vi "LJM logger process data.vi"(6 "Disable Scaling":bool, 9 "Scaling Equation":string[](array[string]), 10 "# Channels":i32, 11 "Voltages":dbl[][](array[numeric]) format="%.3f") -> (0 "error out":errorcluster, 2 "Volts,Scaled Averages":dbl[][](array[numeric]) format="%.3f", 3 "Scaled Data":dbl[][](array[numeric]) format="%.3f")   [LabVIEW 2026]
uses:
  <vilib>/Analysis/baseanly.llb/Mean (DBL).vi
  <vilib>/Analysis/NI_AALBase.lvlib
panel:
  out "First Error":bool
  out "ms":u32
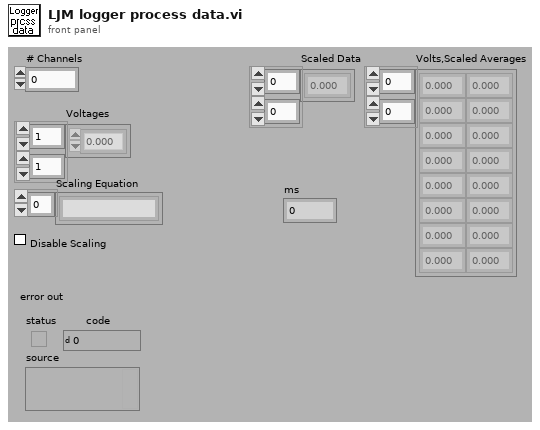
[diagram p1: front panel]
types:
  T1 = typedef "Program Config Cluster.ctl" = cluster{"Data File Prefix":string, "Scan Rate (Hz)":dbl, "Graph History":i32, "# Channels":i32, "Disable Scaling":bool, "Max File Size (Bytes)":i32, "Channel Setup":T2, "Interval (ms)":u32, "Write To File":bool, "Log Every n Scans":i32}
  T2 = typedef "Channel Setup.ctl" = cluster{"Name":string[], string, "Scaling Equation":string[], string, "Graph?":bool[]}
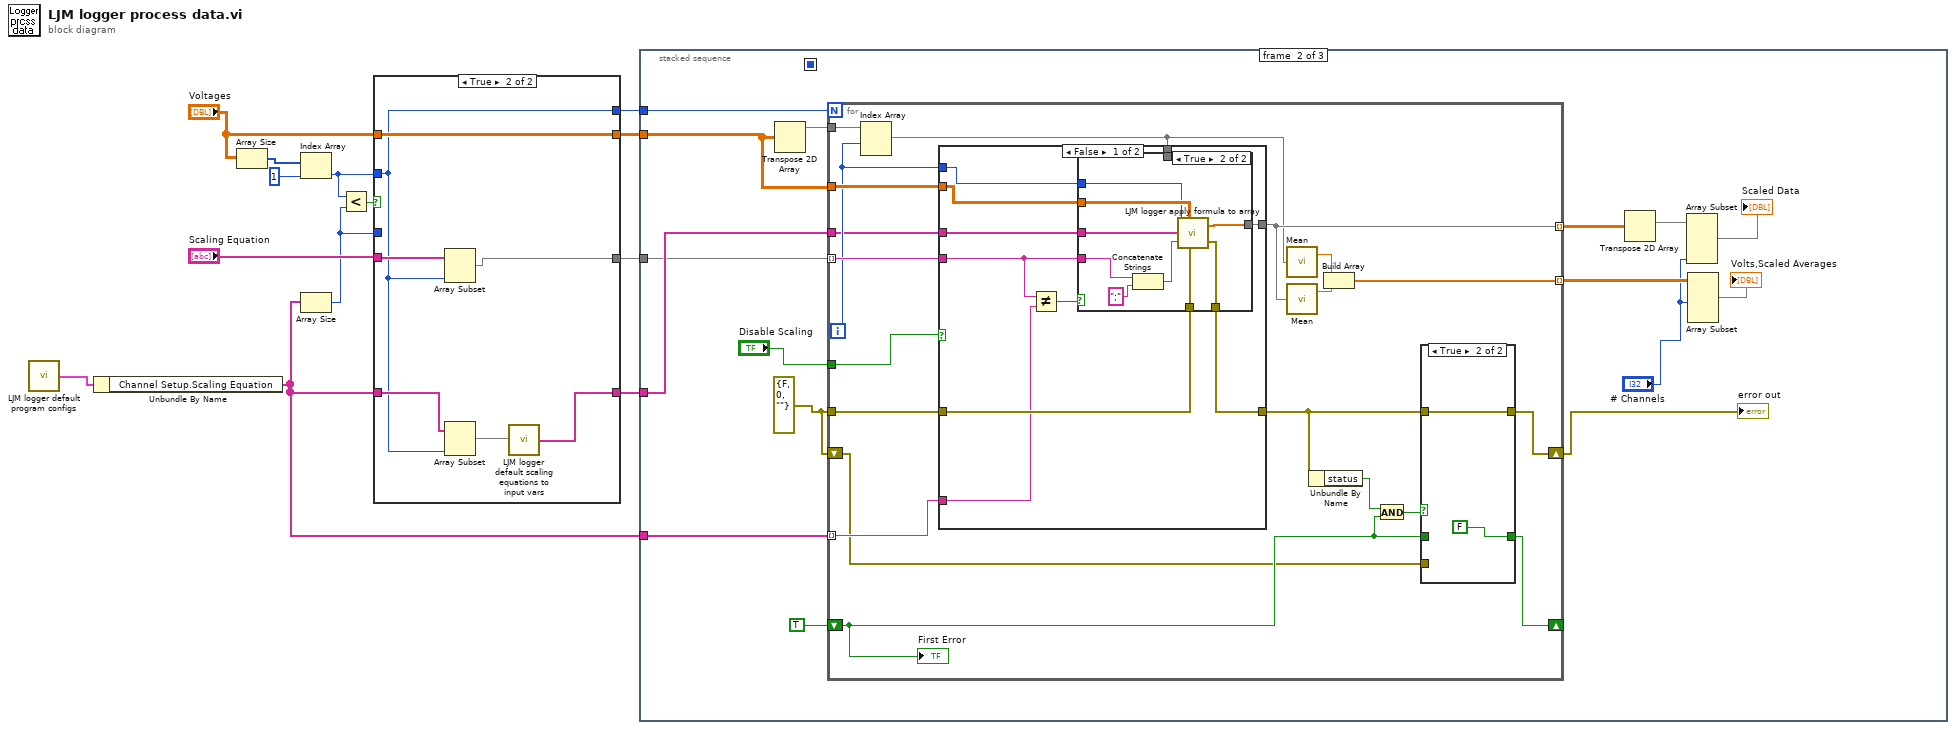
[diagram p0: block diagram]
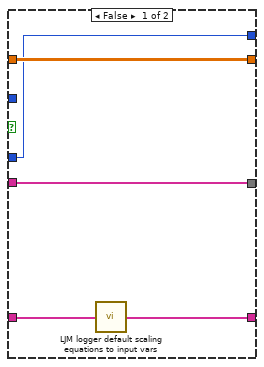
[diagram p2: hidden frame]
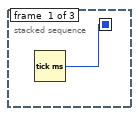
[diagram p3: hidden frame]
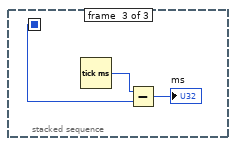
[diagram p7: hidden frame]
diagram:
  n1 = call "LJM logger default program configs.vi"() -> ("Program Configs"=w8:T1)  [unwired: 1 in]
  n2 = Unbundle By Name(w8) -> ("Channel Setup.Scaling Equation"=w4:string[])
  n3 = Array Size(array="Voltages") -> (size(s)=w12:i32[])
  n4 = Index Array(array=w12, index=1 ("Index")) -> (element=w3:i32)
  n5 = Array Size(array=w4) -> (size(s)=w1:i32)
  n6 = Less?(x=w3, y=w1) -> (x < y?=w11:bool)
  n7 = case shown="True" w11 {
    tunnel: w3 -> [_ w19]
    tunnel: "Voltages" -> [w18 w20]
    tunnel: [w18 w20] -> w9
    tunnel: "Scaling Equation" -> [w17 w25]
    tunnel: [w17 w24] -> w6
    tunnel: [w14 w23] -> w5
    tunnel: w4 -> [w15 w21]
    tunnel: [w16 w19] -> w2
    tunnel: w1 -> [w16 _]
    frame False {
      n8 = call "LJM logger default scaling equations to input vars.vi"("Default Scaling Equations"=w15) -> ("Scaling Equation Input Variables"=w14:string[])
    }
    frame True {
      n9 = Array Subset(array=w25, length=w19) -> (w24:string[])  [unwired: 1 in]
      n10 = Array Subset(array=w21, length=w19) -> (w22:string[])  [unwired: 1 in]
      n11 = call "LJM logger default scaling equations to input vars.vi"("Default Scaling Equations"=w22) -> ("Scaling Equation Input Variables"=w23:string[])
    }
  }
  n12 = stacked-sequence {
    seq-local: [w26 _ _] -> [_ _ w91]
    tunnel: w9 -> [_ w40 _]
    tunnel: w4 -> [_ w35 _]
    tunnel: w5 -> [_ w29 _]
    tunnel: w6 -> [_ w28 _]
    tunnel: w2 -> [_ w27 _]
    frame #0 {
      n13 = Tick Count (ms)() -> (millisecond timer value=w26:u32)
    }
    frame #1 {
      w31 = errorcluster {"status"=FALSE, "code"=0, "source"=""} ("error out")
      n14 = Transpose 2D Array(2D array=w40) -> (transposed array=w41:dbl[][])
      n15 = for {
        N: w27 -> [_]
        tunnel: w40 -> [w58]
        tunnel: w28 -> [w57] mode=indexing
        tunnel: [w59] -> w42 mode=indexing
        tunnel: [w60] -> w39 mode=indexing
        tunnel: w41 -> [w56]
        tunnel: w29 -> [w53]
        tunnel: w35 -> [w52] mode=indexing
        tunnel: "Disable Scaling" -> [w51]
        shift-right: [w49] -> _
        shift-left: TRUE ("First Error") -> [w48]
        shift-right: [w45] -> w30
        shift-left: w31 -> [w44]
        tunnel: w31 -> [w50]
        i -> [w54]
        n16 = Index Array(array=w56, index (row)=w54) -> (element=w55:dbl[])  [unwired: 1 in]
        n17 = case shown="False" w51 {
          tunnel: [w76 w89] -> w59
          tunnel: w58 -> [w75 _]
          tunnel: w57 -> [w72 _]
          tunnel: w55 -> [w70 w89]
          tunnel: w54 -> [w74 _]
          tunnel: w53 -> [w73 _]
          tunnel: w52 -> [w67 _]
          tunnel: [w69 w88] -> w46
          tunnel: w50 -> [w68 w88]
          frame False {
            n18 = Not Equal?(x=w72, y=w67) -> (x != y?=w71:bool)
            n19 = case shown="True" w71 {
              tunnel: [w78 w87] -> w76
              tunnel: w75 -> [_ w86]
              tunnel: w74 -> [_ w83]
              tunnel: w73 -> [_ w82]
              tunnel: w72 -> [_ w81]
              tunnel: w70 -> [w78 _]
              tunnel: [w77 w80] -> w69
              tunnel: w68 -> [w77 w79]
              frame False {
              }
              frame True {
                n20 = Concatenate Strings(w81, ";" ("Substring")) -> (w85:string)
                n21 = call "LJM logger apply formula to array.vi"("Index"=w83, "Input Values"=w86, "Variables Input"=w82, "formula"=w85, "error in (no error)"=w79) -> ("Output Values"=w87:dbl[], "error out"=w80:errorcluster)
              }
            }
          }
          frame True {
          }
        }
        n22 = call-poly <vilib>:"Mean.vi"("X"=w55) -> ("mean"=w62:dbl)  [unwired: 1 out]
        n23 = call-poly <vilib>:"Mean.vi"("X"=w59) -> ("mean"=w61:dbl)  [unwired: 1 out]
        n24 = Unbundle By Name(w46) -> ("status"=w43:bool)
        n25 = Build Array(w62, w61) -> (w60:dbl[])
        n26 = And(x=w43, y=w48) -> (x .and. y?=w47:bool)
        n27 = case shown="True" w47 {
          tunnel: w48 -> [w64 _]
          tunnel: [w64 FALSE ("First Error")] -> w49
          tunnel: w46 -> [_ w65]
          tunnel: [w63 w65] -> w45
          tunnel: w44 -> [w63 _]
          frame False {
          }
          frame True {
          }
        }
        "First Error" <- w48
      }
      "error out" <- w30
      n28 = Transpose 2D Array(2D array=w42) -> (transposed array=w37:dbl[][])
      n29 = Array Subset(array=w37, length (col)="# Channels") -> (→"Scaled Data":dbl[][])  [unwired: 3 in]
      n30 = Array Subset(array=w39, length (row)="# Channels") -> (→"Volts,Scaled Averages":dbl[][])  [unwired: 3 in]
    }
    frame #2 {
      n31 = Tick Count (ms)() -> (millisecond timer value=w92:u32)
      n32 = Subtract(x=w92, y=w91) -> (x-y=→"ms":u32)
    }
  }
